vi "AddOperationCycle.vi"(4 "Location (This Machine)":string, 6 "OperationCycleStatus (NOT_COMPLETED)":T1=enum."NOT_COMPLETED", 7 "OperationRunStartTime (Now)":timestamp, 8 "error in":errorcluster, 10 "OperationName (Generic_Operation)":string="Generic_Operation", 11 "ProcessRun in":refnum<class "ProcessRun.lvclass">) -> (0 "error out":errorcluster, 2 "OperationRun":refnum<class "OperationCycle.lvclass">, 3 "ProcessRun out":refnum<class "ProcessRun.lvclass">)   [LabVIEW 2021, in "ProligentXMLGenerator.lvlib" / "ProcessRun.lvclass"]
doc: "Add an OperationRun.\n\nDefines the operation run, a logical container for the execution of sequences and processes.\nOperation runs are globaly unique by their OperationRunId property."
uses:
  ProcessRun.lvclass
  ProcessRun.lvclass/ProcessRun.ctl
  OperationCycle/OperationCycle.lvclass
  ProligentXMLGenerator.lvlib
  Base/ExecutionStatus/Value.ctl
  Base/ExecutionStatus/ExecutionStatus.lvclass
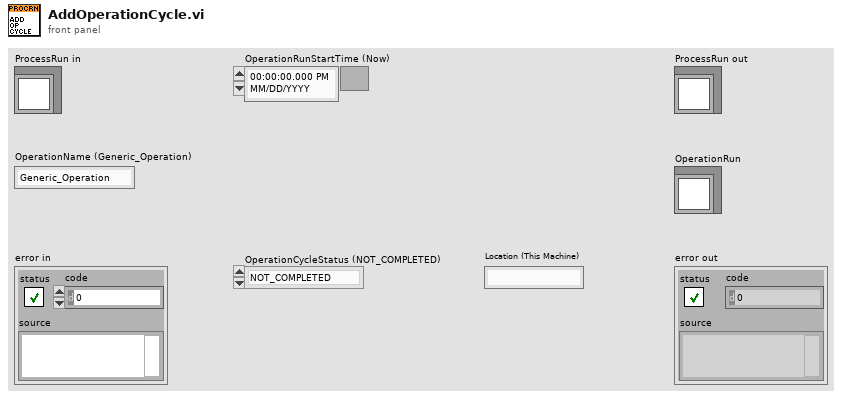
[diagram p1: front panel]
types:
  T1 = typedef "ProligentXMLGenerator.lvlib/ExecutionStatus.lvclass/Value.ctl" = enum16{"PASS", "FAIL", "NOT_COMPLETED", "ABORTED"}
  T2 = typedef "ProligentXMLGenerator.lvlib/ProcessRun.lvclass/Data.ctl" = cluster{"Name":string, "OperationRuns":refnum<class "OperationRun.lvclass">[], "OperationCycles":refnum<class "OperationCycle.lvclass">[], "FailureReferences":refnum<class "FailureReference.lvclass">[], "CustomData":refnum<class "CustomData.lvclass">, "ProcessRunId":refnum<class "Guid.lvclass">, "ProcessFullName":refnum<class "ProcessFullName.lvclass">, "ProcessVersion":refnum<class "NonEmptyString_64.lvclass">, "ProductUnitIdentifier":refnum<class "NonEmptyString_50.lvclass">, "ProductFullName":refnum<class "FullName.lvclass">, "ProcessRunStatus":refnum<class "ExecutionStatus.lvclass">, "ProcessRunStartTime":refnum<class "DateTime.lvclass">, "ProcessRunEndTime":refnum<class "DateTime.lvclass">, "ProcessMode":refnum<class "NonEmptyString_64.lvclass">, "TimeZoneInfoId":string}
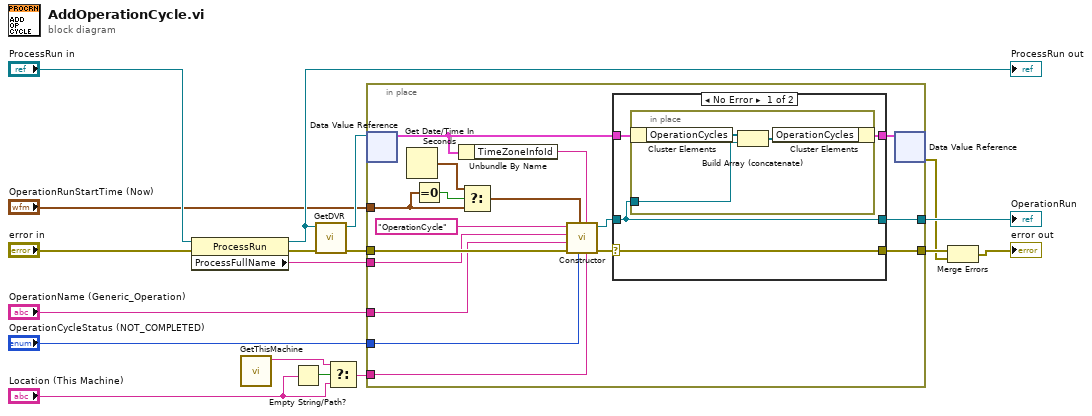
[diagram p0: block diagram]
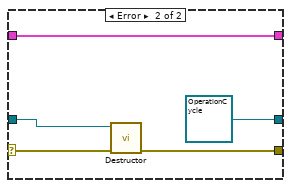
[diagram p2: hidden frame]
diagram:
  n1 = property on="Property Node" class="ProcessRun"(reference="ProcessRun in", error in="error in") -> (reference out=w7:refnum<class "ProcessRun.lvclass">, error out=w9:errorcluster, "ProcessFullName"=w6:string)
  "ProcessRun out" <- w7
  n2 = call "GetThisMachine.vi"() -> ("ThisMachine"=w3:string)  [unwired: 11 in]
  n3 = Empty String/Path?(string/path="Location (This Machine)") -> (empty?=w2:bool)
  n4 = call "GetDVR.vi"("error in"=w9, "ProcessRun"=w7) -> ("error out"=w12:errorcluster, "DVRReference"=w11:refnum<data-value>)  [unwired: 8 in]
  n5 = Select(t=w3, s=w2, f="Location (This Machine)") -> (s? t:f=w4:string)
  n6 = in-place "In Place Element Structure" {
    in-place-border: [w34] -> w13
    in-place-border: w12 -> [w33]
    in-place-border: [w31] -> w16
    in-place-border: "OperationCycleStatus (NOT_COMPLETED)" -> [w27]
    in-place-border: "OperationName (Generic_Operation)" -> [w28]
    in-place-border: w6 -> [w26]
    in-place-border: "OperationRunStartTime (Now)" -> [w23]
    in-place-border: w4 -> [w21]
    n7 = in-place-dvr #1(w11) -> (w20:T2)  [unwired: 1 out]
    n8 = Get Date/Time In Seconds() -> (seconds since 1Jan1904=w24:timestamp)
    n9 = Equal To 0?(x=w23) -> (x = 0?=w25:bool)
    n10 = Unbundle By Name(w20) -> ("TimeZoneInfoId"=w19:string)
    n11 = Select(t=w24, s=w25, f=w23) -> (s? t:f=w22:timestamp)
    n12 = call "Constructor.vi"("Location"=w21, "TimeZoneInfoId"=w19, "OperationCycleStatus"=w27, "OperationCycleStartTime"=w22, "error in"=w33, "OperationName"=w28, "ProcessFullName"=w26, "Name"="OperationCycle") -> ("error out"=w35:errorcluster, "OperationCycle out"=w30:refnum<class "OperationCycle.lvclass">)  [unwired: 2 in]
    n13 = case shown="No Error" w35 {
      selector: w35 -> [w39 w46]
      tunnel: [w36 w47] -> w32
      tunnel: [w39 w45] -> w34
      tunnel: w30 -> [w38 w44]
      tunnel: w20 -> [w37 w47]
      tunnel: [w38 refnum<class "OperationCycle.lvclass"> refnum ("ProligentResultProcessor:OperationCycle")] -> w31
      frame No Error {
        n14 = in-place "In Place Element Structure" {
          in-place-border: w38 -> [w42]
          n15 = in-place-cluster #2(w37) -> ("OperationCycles"=w41:refnum<class "OperationCycle.lvclass">[])
          n16 = Build Array (concatenate)(w41, w42) -> (w40:refnum<class "OperationCycle.lvclass">[])
          n17 = in-place-cluster #2("OperationCycles"=w40) -> (w36:T2)
        }
      }
      frame Error {
        n18 = call "Destructor.vi"("error in"=w46, "OperationCycle in"=w44) -> ("error out"=w45:errorcluster)  [unwired: 9 in]
      }
    }
    n19 = in-place-dvr #1(w32) -> (w10:errorcluster)  [unwired: 1 out]
  }
  "OperationRun" <- w16
  n20 = Merge Errors(w13, w10) -> (→"error out":errorcluster)
